vi "LowLimit.vi"(8 "lower limit":dbl=0.01, 9 "x":dbl, 11 "upper limit":dbl=0.06) -> (1 "out":dbl)   [LabVIEW 2018]
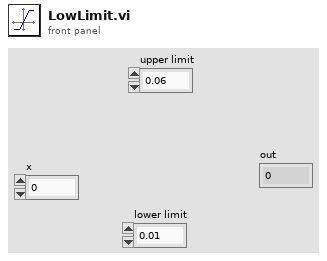
[diagram p1: front panel]
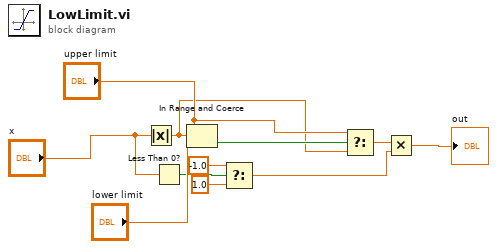
[diagram p0: block diagram]
diagram:
  n1 = Absolute Value(x="x") -> (abs(x)=w4:dbl)
  n2 = Less Than 0?(x="x") -> (x < 0?=w9:bool)
  n3 = In Range and Coerce(upper limit="upper limit", x=w4, lower limit="lower limit") -> (In Range?=w6:bool)  [unwired: 1 out]
  n4 = Select(t=-1.0, s=w9, f=1.0) -> (s? t:f=w2:dbl)
  n5 = Select(t="upper limit", s=w6, f=w4) -> (s? t:f=w3:dbl)
  n6 = Multiply(x=w3, y=w2) -> (x*y=→"out":dbl)
